vi "VisitSites.vi"(0 "Microsites":T2(array[cluster]), 4 "Path":path, 7 "UiDefinition":T1, 13 "CurrentPositionIndex":i32) -> ()   [LabVIEW 2020]
uses:
  UIReferences.ctl
  C:/Users/User/Desktop/Automation/NextVersion2/LabviewDXFViewer/bin/Release/LabviewDXFViewer.exe
  LabviewDXFViewer/bin/Release/LabviewDXFViewer.exe
  <vilib>/Utility/file.llb/Write Delimited Spreadsheet (string).vi
  <vilib>/Utility/file.llb/Write Delimited Spreadsheet (DBL).vi
panel:
  out "error out":errorcluster
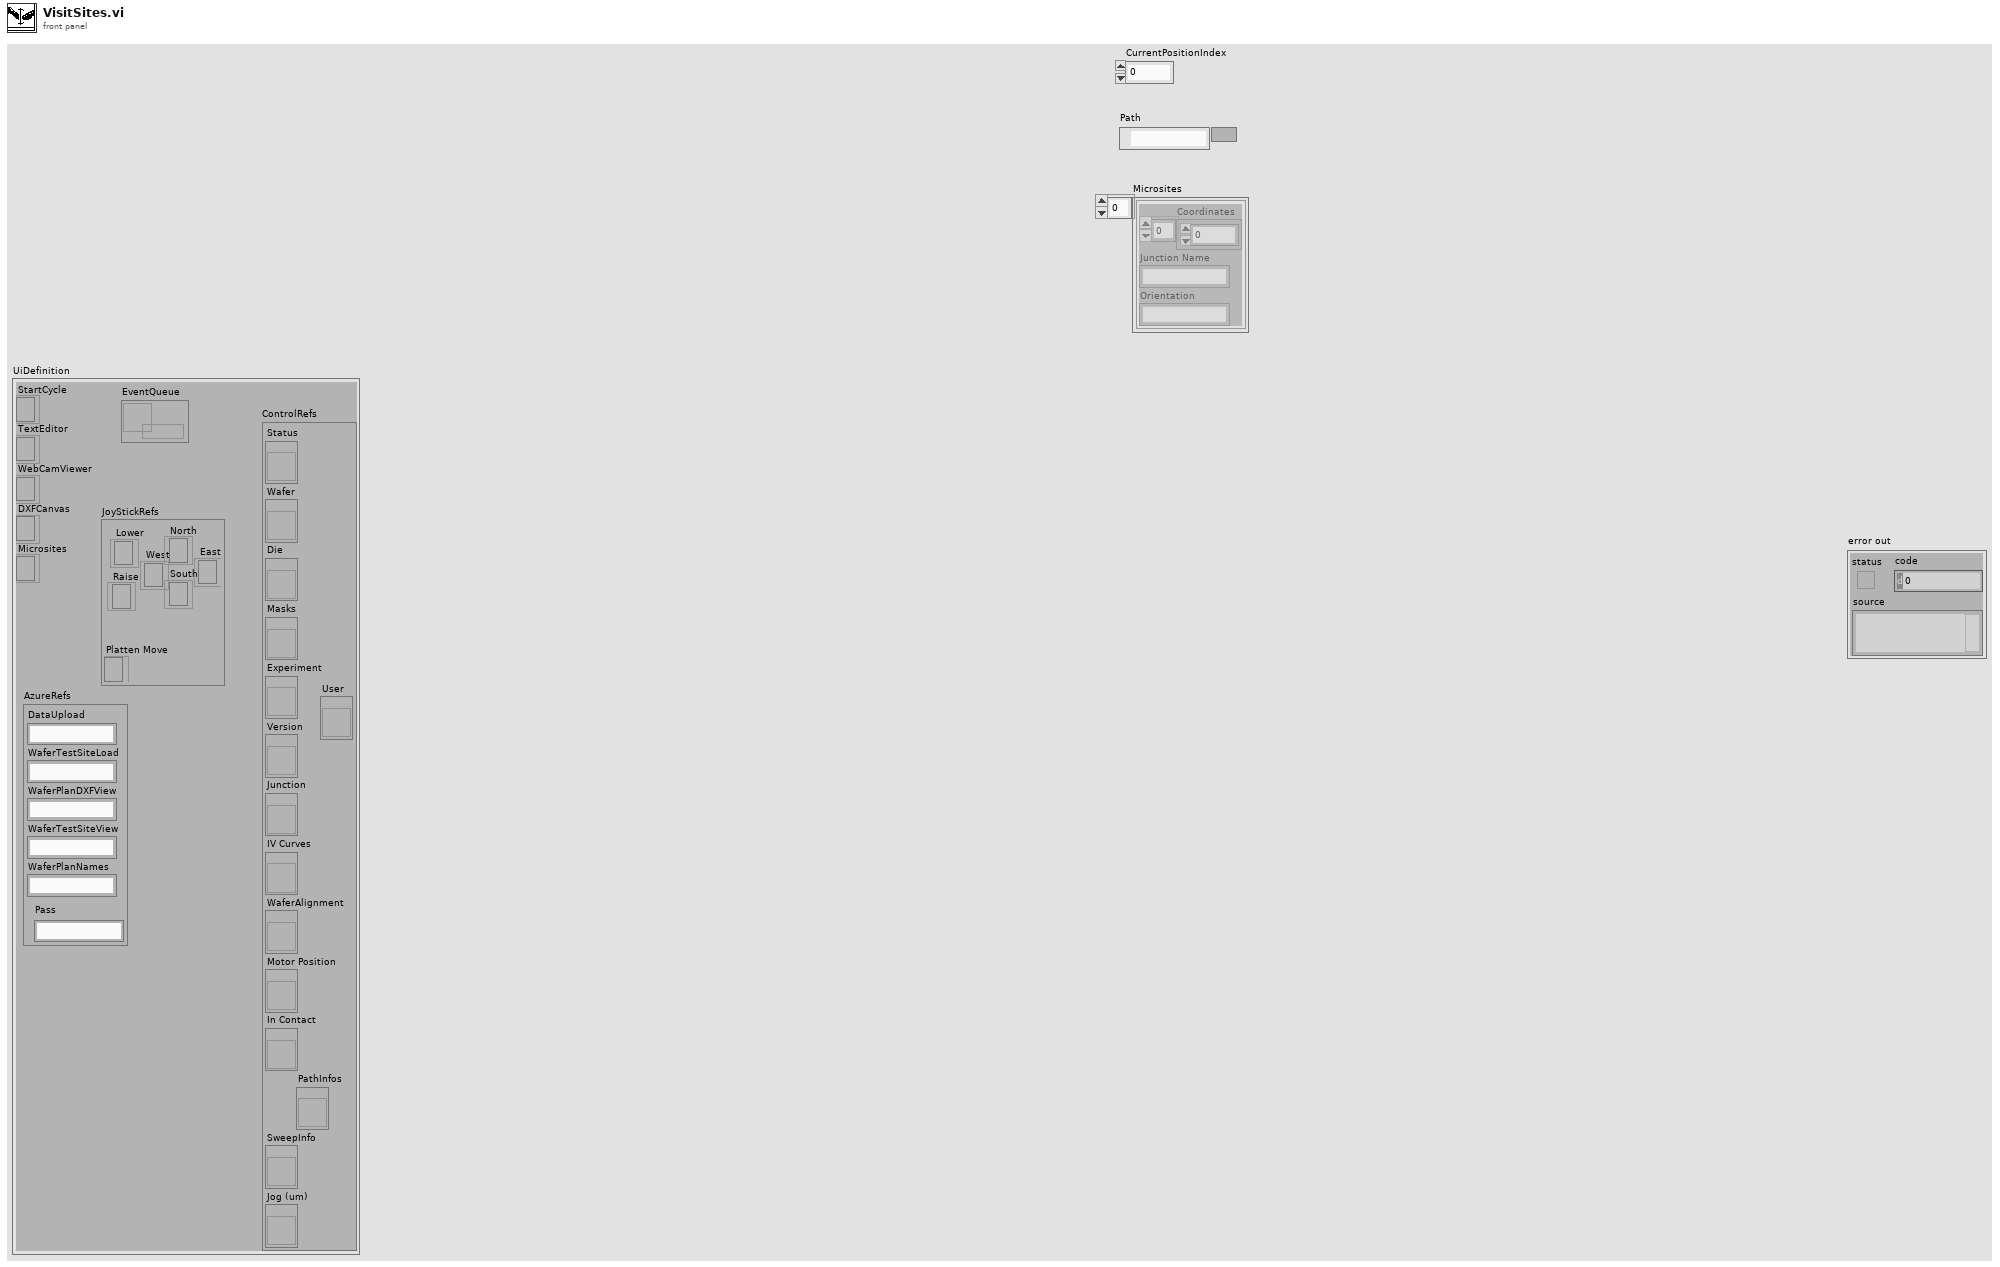
[diagram p1: front panel]
types:
  T1 = typedef "UIReferences.ctl" = cluster{"StartCycle":refnum<k24>, "TextEditor":refnum<k24>, "WebCamViewer":refnum<k24>, "DXFCanvas":refnum<k24>, "Microsites":refnum<k24>, "JoyStickRefs":cluster{"North":refnum<k24>, "Lower":refnum<k24>, "Raise":refnum<k24>, "Platten Move":refnum<k24>, "West":refnum<k24>, "East":refnum<k24>, "South":refnum<k24>}, "AzureRefs":cluster{"DataUpload":string, "WaferTestSiteLoad":string, "WaferPlanDXFView":string, "WaferTestSiteView":string, "WaferPlanNames":string, "Pass":string}, "ControlRefs":cluster{"Status":refnum<vi>, "Wafer":refnum<vi>, "Die":refnum<vi>, "Masks":refnum<vi>, "Experiment":refnum<vi>, "Version":refnum<vi>, "Junction":refnum<vi>, "IV Curves":refnum<vi>, "WaferAlignment":refnum<vi>, "Motor Position":refnum<vi>, "In Contact":refnum<vi>, "SweepInfo":refnum<vi>, "Jog (um)":refnum<vi>, "PathInfos":refnum<vi>, "User":refnum<vi>}, "EventQueue":refnum<queue>}
  T2 = cluster{"Coordinates":dbl[], "Junction Name":string, "Orientation":string}[]
  T3 = cluster{"Coordinates":dbl[], "Junction Name":string, "Orientation":string}
  T4 = cluster{"Wafer Units to microns":dbl, "Rotation Misalign":dbl[], "Scale Misalign":dbl, "Steps Per micron":dbl, "Position 1":i32[], "Chip Orientation":i32, "Position 2":i32[], "Lift Distance":i32, "Position 3":i32[]}
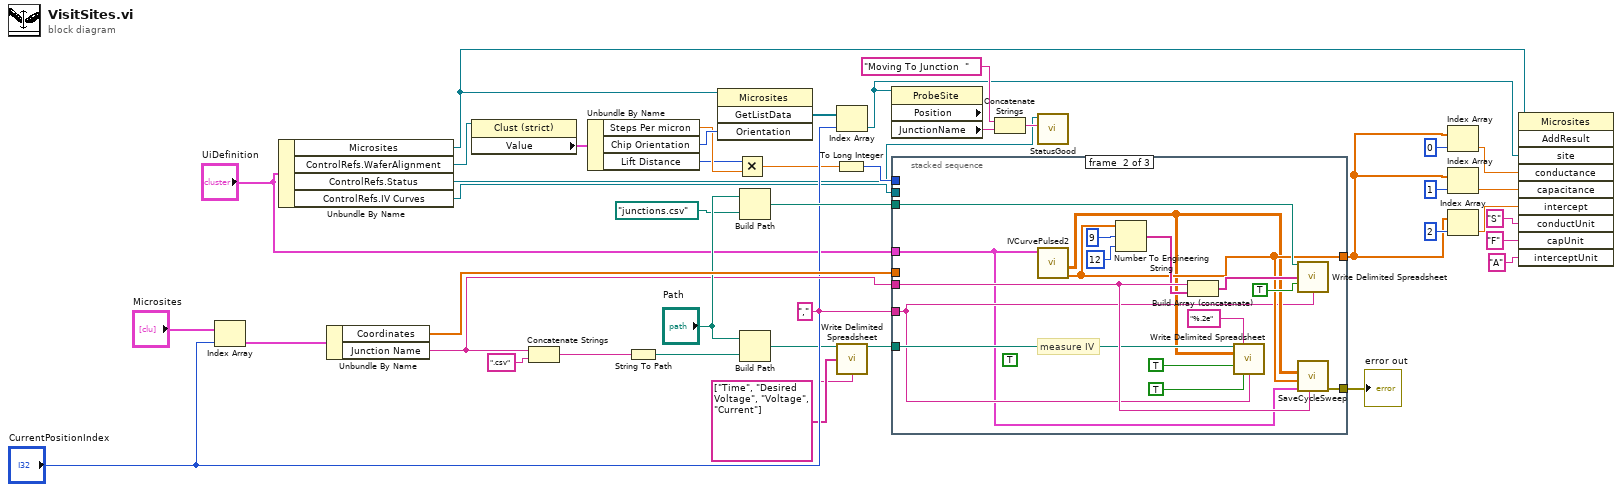
[diagram p0: block diagram]
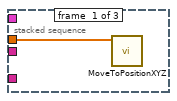
[diagram p2: hidden frame]
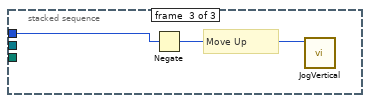
[diagram p3: hidden frame]
diagram:
  w9 = "," ("delimiter (\\t)")
  n1 = Index Array(array="Microsites", index="CurrentPositionIndex") -> (element=w32:T3)
  n2 = Unbundle By Name("UiDefinition") -> ("Microsites"=w8:refnum<k24>, "ControlRefs.WaferAlignment"=w26:refnum<vi>, "ControlRefs.Status"=w23:refnum<vi>, "ControlRefs.IV Curves"=w18:refnum<vi>)
  n3 = Unbundle By Name(w32) -> ("Coordinates"=w40:dbl[], "Junction Name"=w34:string)
  n4 = property class="Clust (strict)"(reference=w26) -> ("Value"=w25:T4)  [unwired: 1 in, 2 out]
  n5 = Concatenate Strings(w34, ".csv" ("string")) -> (w39:string)
  n6 = Unbundle By Name(w25) -> ("Steps Per micron"=w21:dbl, "Chip Orientation"=w24:i32, "Lift Distance"=w20:i32)
  n7 = String To Path(string=w39) -> (path=w38:path)
  n8 = invoke class="Microsites" method="GetListData"(reference=w8, "Orientation"=w24) -> ("GetListData"=w27:refnum<k24>[])  [unwired: 2 in, 3 out]
  n9 = Multiply(x=w20, y=w21) -> (x*y=w22:dbl)
  n10 = Build Path(base path="Path", name or relative path=path "junctions.csv") -> (appended path=w41:path)
  n11 = Build Path(base path="Path", name or relative path=w38) -> (appended path=w12:path)
  n12 = To Long Integer(number=w22) -> (32bit integer=w42:i32)
  n13 = Index Array(array=w27, index="CurrentPositionIndex") -> (element=w7:refnum<k24>)
  n14 = call-poly <vilib>:"Write Delimited Spreadsheet.vi"("file path (dialog if empty)"=w12, "1D data"=string[] ["Time", "Desired Voltage", "Voltage", "Current"], "delimiter (\\t)"=w9) -> ("new file path (Not A Path if cancelled)"=w10:path)  [unwired: 11 in, 1 out]
  n15 = property class="ProbeSite" props=["Position", "JunctionName"](reference=w7) -> ("JunctionName"=w31:string)  [unwired: 1 in, 3 out]
  n16 = stacked-sequence {
    tunnel: w42 -> [_ _ w61]
    tunnel: w41 -> [_ w59 _]
    tunnel: w40 -> [w43 _ _]
    tunnel: w34 -> [_ w58 _]
    tunnel: w10 -> [_ w57 _]
    tunnel: w18 -> [_ _ _]
    tunnel: "UiDefinition" -> [_ w44 _]
    tunnel: [_ w49 _] -> w16
    tunnel: [_ w48 _] -> w13
    tunnel: w9 -> [_ w45 _]
    frame #0 {
      n17 = call "MoveToPositionXYZ.vi"("Array"=w43) -> ()  [unwired: 11 in]
    }
    frame #1 {
      (unwired) TRUE ("Reprogram")
      # "measure IV"
      n18 = call "IVCurvePulsed2.vi"("UiDefinition"=w44) -> ("Fit 2"=w48:dbl[], "appended array"=w47:dbl[][])  [unwired: 9 in]
      n19 = Number To Engineering String(2:i16 12 ("precision (6)"), 3:i16 9 ("width (-)"), 4:w48) -> (0:w55:string[])  [unwired: 1 in]
      n20 = Build Array (concatenate)(w58, w55) -> (w53:string[])
      n21 = call-poly <vilib>:"Write Delimited Spreadsheet.vi"("file path (dialog if empty)"=w57, "format (%.3f)"="%.2e", "2D data"=w47, "append to file? (new file:F)"=TRUE, "transpose? (no:F)"=TRUE, "delimiter (\\t)"=w45) -> ()  [unwired: 8 in, 2 out]
      n22 = call-poly <vilib>:"Write Delimited Spreadsheet.vi"("file path (dialog if empty)"=w59, "1D data"=w53, "append to file? (new file:F)"=TRUE, "delimiter (\\t)"=w45) -> ()  [unwired: 10 in, 2 out]
      n23 = call "SaveCycleSweep.vi"("JunctionName"=w58, "UiDefinition 2"=w44, "Fit in"=w48, "appended array"=w47) -> ("error out"=w49:errorcluster)  [unwired: 7 in]
    }
    frame #2 {
      # "Move Up"
      n24 = Negate(x=w61) -> (-x=w60:i32)
      n25 = call "JogVertical.vi"("Numeric"=w60) -> ()  [unwired: 11 in]
    }
  }
  "error out" <- w16
  n26 = Concatenate Strings("Moving To Junction  " ("Text.Text"), w31) -> (w30:string)
  n27 = call "StatusGood.vi"("Text.Text"=w30, "String in"=w23) -> ()  [unwired: 10 in]
  n28 = Index Array(array=w13, index=0) -> (element=w6:dbl)
  n29 = Index Array(array=w13, index=1) -> (element=w5:dbl)
  n30 = Index Array(array=w13, index=2) -> (element=w4:dbl)
  n31 = invoke class="Microsites" method="AddResult"(reference=w8, "site"=w7, "conductance"=w6, "capacitance"=w5, "intercept"=w4, "conductUnit"="S", "capUnit"="F", "interceptUnit"="A") -> ()  [unwired: 2 in, 10 out]
